vi "DoubleToUInt.vi"(1 "Value":dbl=-327.68, 2 "Max":dbl=327.67, 3 "Min":dbl=-327.68) -> (0 "scaled Integer":u32)   [LabVIEW 2009]
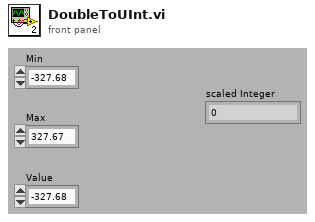
[diagram p1: front panel]
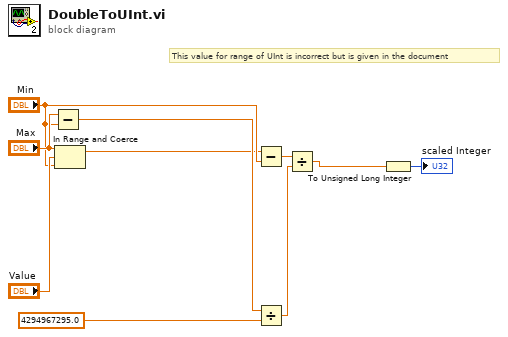
[diagram p0: block diagram]
diagram:
  # "This value for range of UInt is incorrect but is given in the document"
  n1 = Subtract(x="Max", y="Min") -> (x-y=w10:dbl)
  n2 = In Range and Coerce(upper limit="Max", x="Value", lower limit="Min") -> (coerced(x)=w3:dbl)  [unwired: 1 out]
  n3 = Subtract(x=w3, y="Min") -> (x-y=w2:dbl)
  n4 = Divide(x=w10, y=4294967295.0) -> (x/y=w7:dbl)
  n5 = Divide(x=w2, y=w7) -> (x/y=w1:dbl)
  n6 = To Unsigned Long Integer(number=w1) -> (unsigned 32bit integer=→"scaled Integer":u32)
